vi "Time2Sec.vi"(11 "Total Duration":timestamp) -> (3 "Numeric":i32)   [LabVIEW 2018]
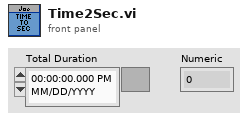
[diagram p1: front panel]
types:
  T1 = typedef "LVDateTimeRec.ctl" = cluster{"fractional second":dbl, "second":i32, "minute":i32, "hour":i32, "day of month":i32, "month":i32, "year":i32, "day of week":i32, "day of year":i32, "DST":i32}
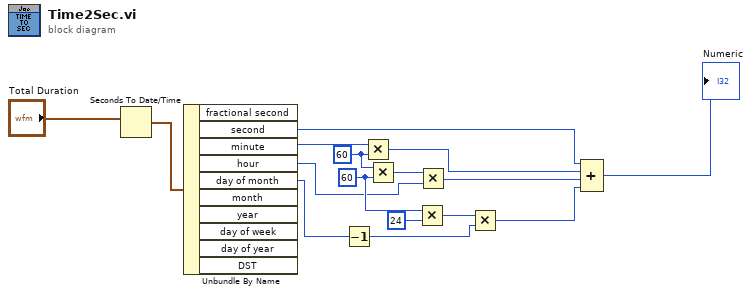
[diagram p0: block diagram]
diagram:
  w7 = 60 ("y")
  w4 = 60 ("y")
  n1 = Seconds To Date/Time(time stamp (now)="Total Duration") -> (date time rec=w2:T1)  [unwired: 1 in]
  n2 = Unbundle By Name(w2) -> ("second"=w11:i32, "minute"=w3:i32, "hour"=w6:i32, "day of month"=w10:i32)  [unwired: 6 out]
  n3 = Decrement(x=w10) -> (x-1=w15:i32)
  n4 = Multiply(x=w3, y=w4) -> (x*y=w12:i32)
  n5 = Multiply(x=w4, y=w7) -> (x*y=w5:i32)
  n6 = Multiply(x=w7, y=24) -> (x*y=w9:i32)
  n7 = Multiply(x=w5, y=w6) -> (x*y=w13:i32)
  n8 = Multiply(x=w9, y=w15) -> (x*y=w14:i32)
  n9 = Compound Arithmetic op=ADD(w11, w12, w13, w14) -> (→"Numeric":i32)
